vi "Go To Absolute Position.vi"(4 "dwell time":u32, 5 "rotate?":T1, 6 "magnification":T2 items=["0.63"=0.63, ".8"=0.8, "1"=1.0, "1.25"=1.25, "1.6"=1.6, "2"=2.0, "2.5"=2.5, "3.2"=3.2, "4"=4.0], 7 "Step":u8(slide) scale=0.0..3.0, 8 "error in":errorcluster, 9 "offset true position":dbl[](array[numeric]), 10 "new position":dbl[](array[numeric]), 11 "Visa Array In":refnum<visa-resource-name>[](array[refnum])) -> (0 "error out":errorcluster, 3 "Visa Array Out":refnum<visa-resource-name>[](array[refnum]))   [LabVIEW 2010, in "SignalWriterMH110203USBStepperMotor.lvclass"]
uses:
  SignalWriterMH110203USBStepperMotor.lvclass
  zoom_controller.ctl
  rotate_controller.ctl
  class_data.vi
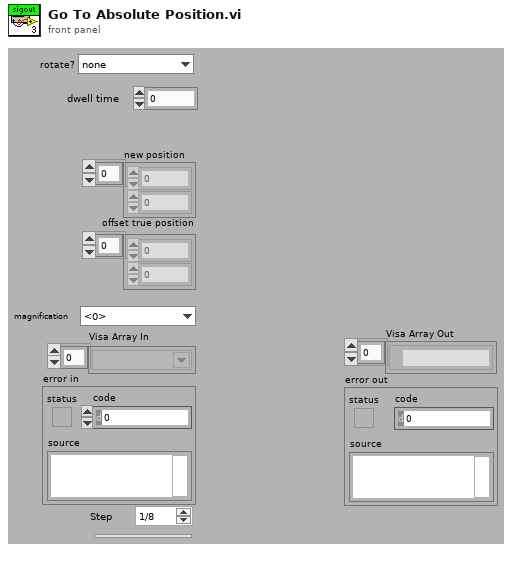
[diagram p1: front panel]
types:
  T1 = typedef "SignalWriterMH110203USBStepperMotor.lvclass/rotate_controller.ctl" = enum16{"none", "90", "180", "270", "mirror horizontal"}
  T2 = typedef "SignalWriterMH110203USBStepperMotor.lvclass/zoom_controller.ctl" = dbl
  T3 = typedef "SignalWriterMH110203USBStepperMotor.lvclass/GoTo Control (uSMC).ctl" = cluster{"Step motor ID":string, "SMname":string, "Backlash":u16, "wait for input sygnal to start":bool, "use slow start/stop":bool, "units name":string, "Maximum speed":dbl, "speed":dbl, "step":u8, "point 1 ticks":i32, "point 2 ticks":i32, "point 1 units":dbl, "point 2 units":dbl, "Limit Switch standoff":dbl, "Zero Value":dbl, "Destination Position":dbl, "force backlash":bool, "power off when stop":bool, "POff delay":dbl, "positioner name":string, "R, Ohm":dbl, "I, mA":dbl, "Positioner's Type":u16, "Reset Direction":bool, "Manufacturer":string, "Model":string, "Scheme":string, "FirmwareVer":string}
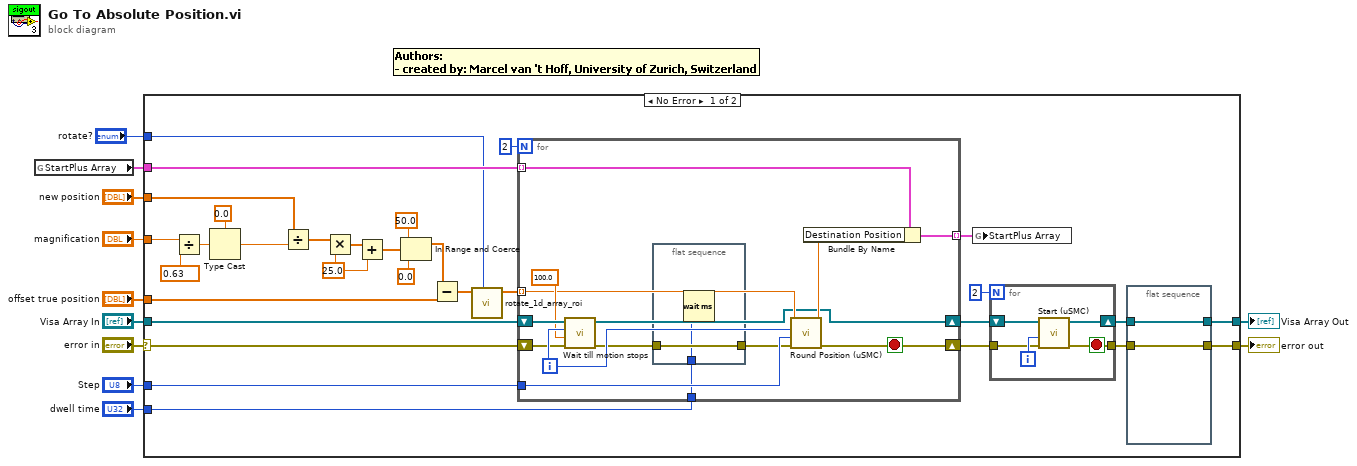
[diagram p0: block diagram]
diagram:
  n1 = global read "class_data.vi" "StartPlus Array"() -> (w11:T3[])
  n2 = case shown="No Error" "error in" {
    selector: "error in" -> [w35 w67]
    tunnel: w11 -> [w37 _]
    tunnel: [w18 w67] -> w10
    tunnel: "Step" -> [w40 _]
    tunnel: [w17 w66] -> w7
    tunnel: "Visa Array In" -> [w36 w66]
    tunnel: "new position" -> [w22 _]
    tunnel: "offset true position" -> [w33 _]
    tunnel: "magnification" -> [w30 _]
    tunnel: "dwell time" -> [w15 _]
    tunnel: "rotate?" -> [w12 _]
    frame No Error {
      w25 = 25.0
      w31 = T2 0.63 items=["0.63"=0.63, ".8"=0.8, "1"=1.0, "1.25"=1.25, "1.6"=1.6, "2"=2.0, "2.5"=2.5, "3.2"=3.2, "4"=4.0] ("y")
      n3 = Divide(x=w30, y=w31) -> (x/y=w29:T2)
      n4 = Type Cast(type=0.0 ("Position(rounded)"), x=w29) -> (*(type *) &x=w23:dbl)
      n5 = Divide(x=w22, y=w23) -> (x/y=w21:dbl[])
      n6 = Multiply(x=w21, y=w25) -> (x*y=w28:dbl[])
      n7 = Add(x=w28, y=w25) -> (x+y=w27:dbl[])
      n8 = In Range and Coerce(upper limit=50.0, x=w27, lower limit=0.0) -> (coerced(x)=w20:dbl[])  [unwired: 1 out]
      n9 = Subtract(x=w20, y=w33) -> (x-y=w14:dbl[])
      n10 = call "rotate_1d_array_roi.vi"("rotate?"=w12, "array in"=w14) -> ("array out"=w13:dbl[])  [unwired: 9 in]
      n11 = for {
        N: 2 -> [_]
        tunnel: w37 -> [w55] mode=indexing
        tunnel: [w54] -> w34 mode=indexing
        tunnel: w40 -> [w57]
        tunnel: w13 -> [w49] mode=indexing
        shift-right: [w48] -> w38
        shift-left: w36 -> [w53]
        shift-right: [w56] -> w39
        shift-left: w35 -> [w51]
        tunnel: w15 -> [w45]
        i -> [w52]
        stop <- w56 stop-if-true
        n12 = call "Wait till motion stops.vi"("error in"=w51, "Timeout (sec)"=100.0, "Index"=w52, "Visa Array Out"=w53) -> ("error out"=w47:errorcluster, "Visa array out"=w48:refnum<visa-resource-name>[])  [unwired: 4 in, 2 out]
        n13 = flat-sequence {
          tunnel: [w60] -> w46
          tunnel: w47 -> [w60]
          tunnel: w45 -> [w59]
          frame #0 {
            n14 = Wait (ms)(milliseconds to wait=w59) -> ()  [unwired: 1 out]
          }
        }
        n15 = call "Round Position (uSMC).vi"("error in"=w46, "Step"=w57, "index"=w52, "Position(value)"=w49) -> ("error out"=w56:errorcluster, "Position(rounded)"=w58:dbl)  [unwired: 6 in]
        n16 = Bundle By Name(cluster=w55, "Destination Position"=w58) -> (w54:T3)
      }
      n17 = global write "class_data.vi" "StartPlus Array"(w34) -> ()
      n18 = for {
        N: 2 -> [_]
        tunnel: w39 -> [w62]
        tunnel: [w61] -> w19
        shift-right: [w64] -> w16
        shift-left: w38 -> [w65]
        i -> [w63]
        stop <- w61 stop-if-true
        n19 = call "Start (uSMC).vi"("error in"=w62, "Index"=w63, "Visa Array In"=w65) -> ("error out"=w61:errorcluster, "Visa Array Out"=w64:refnum<visa-resource-name>[])  [unwired: 7 in]
      }
      n20 = flat-sequence {
        tunnel: [w44] -> w18
        tunnel: w19 -> [w44]
        tunnel: [w43] -> w17
        tunnel: w16 -> [w43]
        frame #0 {
        }
      }
    }
    frame Error {
    }
  }
  "error out" <- w10
  "Visa Array Out" <- w7
